vi "SetVerticalArrangement__slk_mt.vi"(8 "error in (no error)":errorcluster, 11 "label in":refnum<class "Label__slk_mt.lvclass">) -> (0 "error out":errorcluster, 3 "label out":refnum<class "Label__slk_mt.lvclass">)   [LabVIEW 2011, in "Lazyboots Menu Tool.lvlib" / "Label__slk_mt.lvclass"]
doc: "Sets vertical arrangement of label object."
uses:
  Label__slk_mt.lvclass
  Label__slk_mt.lvclass/Label__slk_mt.ctl
  Segment/Segment__slk_mt.lvclass
panel:
  # "SetVerticalArrangement__slk_mt.vi\nSets vertical arrangement of label object.\n\nNOTICE -- YOU MUST LEAVE THIS NOTICE IN PLACE.\n\nCopyright (c) 2011, LIANG LIU Shawn.Liu.cn@gmail.com\nAll rights reserved.\n\nRedistribution and use in source and binary forms, with or without modification, are permitted provided that the following conditions are met:\n-Redistributions of source code must retain the above copyright notice, this list of conditions and the following disclaimer.\n-Redistributions in binary form must reproduce the above copyright notice, this list of conditions and the following disclaimer in the documentation and/or other materials provided with the distribution.\n-Neither the name of the eLp nor the names of its contributors may be used to endorse or promote products derived from this software without specific prior written permission.\n\nTHIS SOFTWARE IS PROVIDED BY THE COPYRIGHT HOLDERS AND CONTRIBUTORS \"AS IS\" AND ANY EXPRESS OR IMPLIED WARRANTIES, INCLUDING, BUT NOT LIMITED TO, THE IMPLIED WARRANTIES OF MERCHANTABILITY AND FITNESS FOR A PARTICULAR PURPOSE ARE DISCLAIMED. IN NO EVENT SHALL THE COPYRIGHT HOLDER OR CONTRIBUTORS BE LIABLE FOR ANY DIRECT, INDIRECT, INCIDENTAL, SPECIAL, EXEMPLARY, OR CONSEQUENTIAL DAMAGES (INCLUDING, BUT NOT LIMITED TO, PROCUREMENT OF SUBSTITUTE GOODS OR SERVICES; LOSS OF USE, DATA, OR PROFITS; OR BUSINESS INTERRUPTION) HOWEVER CAUSED AND ON ANY THEORY OF LIABILITY, WHETHER IN CONTRACT, STRICT LIABILITY, OR TORT (INCLUDING NEGLIGENCE OR OTHERWISE) ARISING IN ANY WAY OUT OF THE USE OF THIS SOFTWARE, EVEN IF ADVISED OF THE POSSIBILITY OF SUCH DAMAGE."
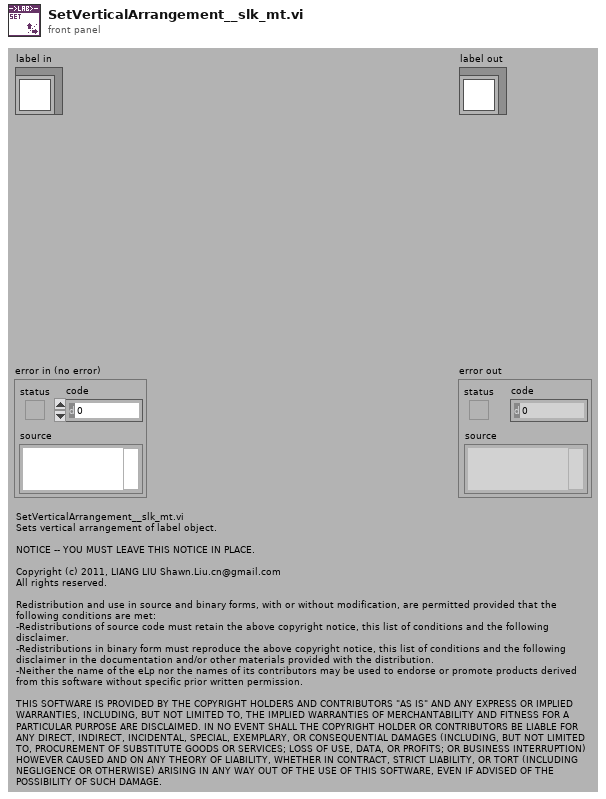
[diagram p1: front panel]
types:
  T1 = enum16{"None", "Stacked", "Clockwise", "Counterclockwise"}
  T2 = typedef "Lazyboots Menu Tool.lvlib/TypeDef_Direction__slk_mt.ctl" = enum16{"Rightward", "Leftward", "Downward", "Upward"}
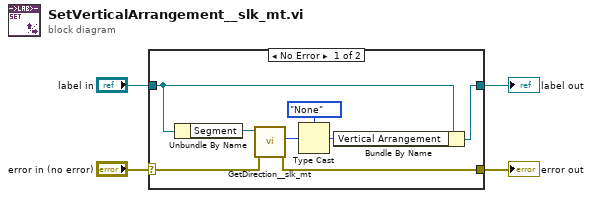
[diagram p0: block diagram]
diagram:
  n1 = case shown="No Error" "error in (no error)" {
    selector: "error in (no error)" -> [w8 w13]
    tunnel: [w7 w13] -> w3
    tunnel: [w12 w14] -> w1
    tunnel: "label in" -> [w6 w14]
    frame No Error {
      n2 = Unbundle By Name(w6) -> ("Segment"=w5:refnum<class "Segment__slk_mt.lvclass">)
      n3 = call "GetDirection__slk_mt.vi"("error in (no error)"=w8, "segment in"=w5) -> ("error out"=w7:errorcluster, "direction"=w11:T2)  [unwired: 7 in, 1 out]
      n4 = Type Cast(type=T1."None" ("Vertical Arrangement"), x=w11) -> (*(type *) &x=w9:T1)
      n5 = Bundle By Name(cluster=w6, "Vertical Arrangement"=w9) -> (w12:refnum<class "Label__slk_mt.lvclass">)
    }
    frame Error {
    }
  }
  "error out" <- w3
  "label out" <- w1
